vi "Aim.vi"() -> ()   [LabVIEW 2017]
panel:
  out "distance error":dbl
  in  "kp Distance":dbl=-0.1
  out "distance adjust":dbl
  in  "ty":dbl=0.6
  in  "tv":dbl=1.0
  in  "Minimum command":dbl=0.05
  out "heading error":dbl
  out "steering adjust":dbl
  out "Right command":dbl
  out "left command":dbl
  in  "kp Aim":dbl=-0.1
  in  "tx":dbl=1.2
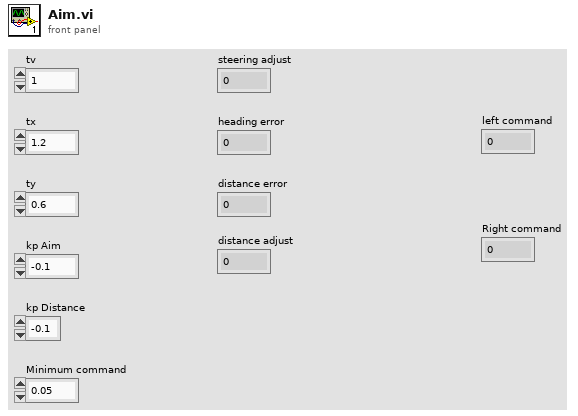
[diagram p1: front panel]
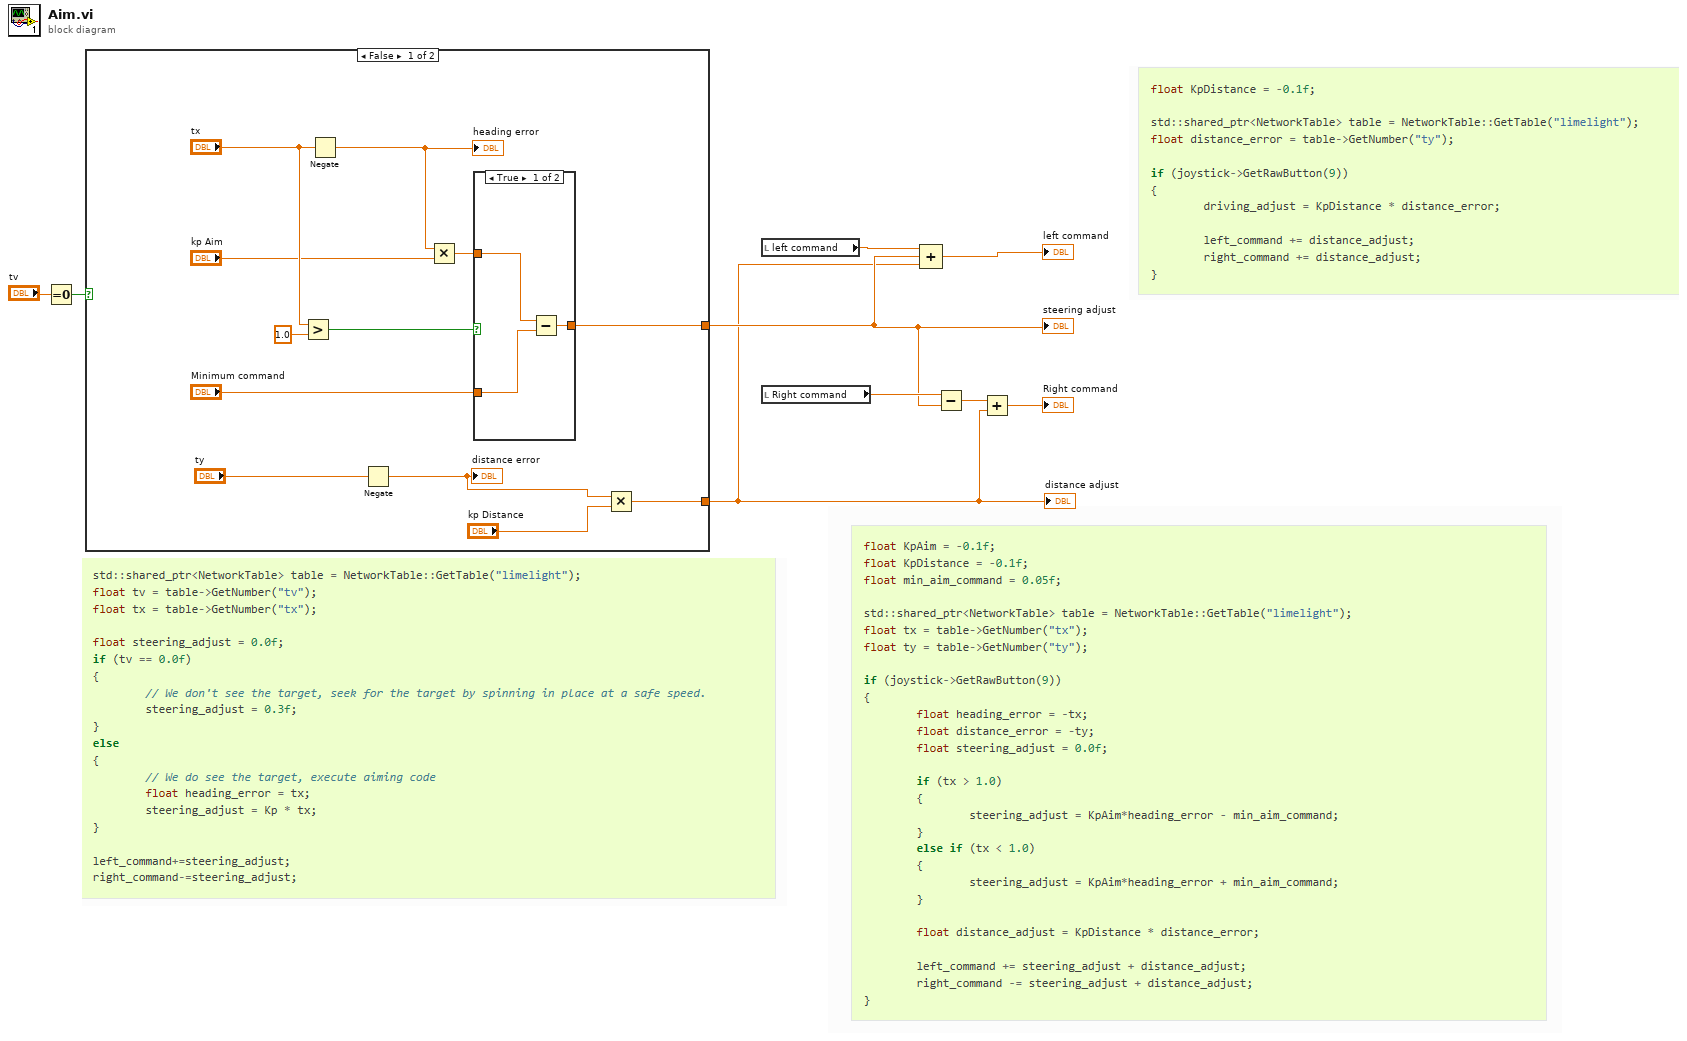
[diagram p0: block diagram]
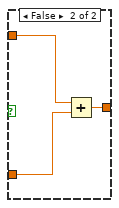
[diagram p2: hidden frame]
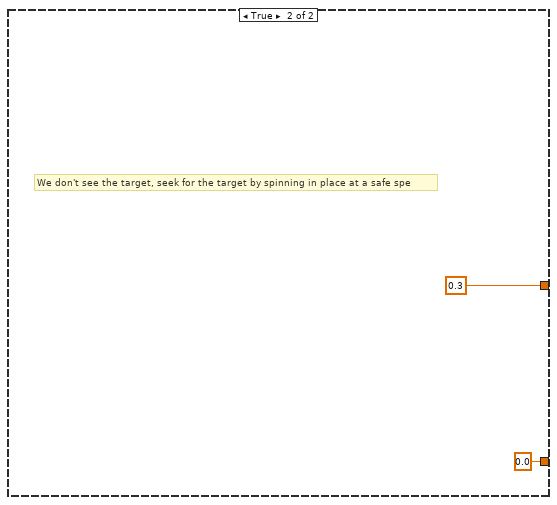
[diagram p3: hidden frame]
diagram:
  n1 = Equal To 0?(x="tv") -> (x = 0?=w8:bool)
  n2 = case shown="False" w8 {
    tunnel: [w14 0.3] -> w4
    tunnel: [w10 0.0] -> w3
    frame False {
      n3 = Greater?(x="tx", y=1.0) -> (0:w21:bool)
      n4 = Negate(x="tx") -> (-x=w18:dbl)
      "heading error" <- w18
      n5 = Negate(x="ty") -> (-x=w12:dbl)
      "distance error" <- w12
      n6 = Multiply(x=w18, y="kp Aim") -> (x*y=w16:dbl)
      n7 = case shown="True" w21 {
        tunnel: w16 -> [w24 w27]
        tunnel: "Minimum command" -> [w23 w26]
        tunnel: [w22 w25] -> w14
        frame True {
          n8 = Subtract(x=w24, y=w23) -> (x-y=w22:dbl)
        }
        frame False {
          n9 = Add(x=w27, y=w26) -> (x+y=w25:dbl)
        }
      }
      n10 = Multiply(x=w12, y="kp Distance") -> (x*y=w10:dbl)
    }
    frame True {
      # "We don't see the target, seek for the target by spinning in place at a safe spe"
    }
  }
  "steering adjust" <- w4
  "distance adjust" <- w3
  n11 = local read "left command"() -> (w6:dbl)
  n12 = local read "Right command"() -> (w7:dbl)
  n13 = Compound Arithmetic op=ADD(w6, w4, w3) -> (→"left command":dbl)
  n14 = Subtract(x=w7, y=w4) -> (x-y=w2:dbl)
  n15 = Add(x=w2, y=w3) -> (x+y=→"Right command":dbl)
